vi "RadiusOfCircleThreePoints.vi"(11 "Points":cluster{"X":dbl, "Y":dbl}[](array[cluster])) -> (3 "R":dbl)   [LabVIEW 2017]
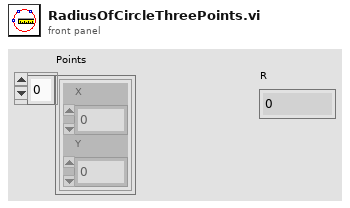
[diagram p1: front panel]
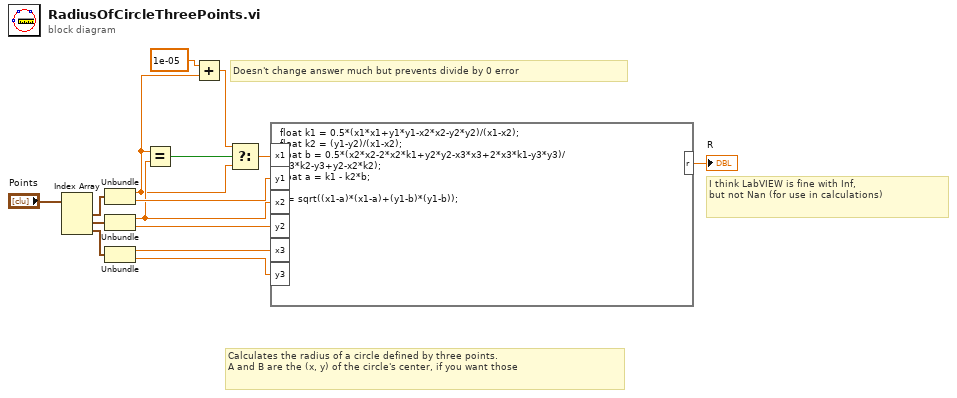
[diagram p0: block diagram]
diagram:
  # "Calculates the radius of a circle defined by three points.\nA and B are the (x, y) of the circle's center, if you want those"
  # "I think LabVIEW is fine with Inf,\nbut not Nan (for use in calculations)"
  # "Doesn't change answer much but prevents divide by 0 error"
  n1 = Index Array(array="Points") -> (element #1=w3:cluster{"X":dbl, "Y":dbl}, element #2=w2:cluster{"X":dbl, "Y":dbl}, element #3=w1:cluster{"X":dbl, "Y":dbl})  [unwired: 3 in]
  n2 = Unbundle(w3) -> ("X"=w8:dbl, "Y"=w15:dbl)
  n3 = Unbundle(w2) -> ("X"=w11:dbl, "Y"=w14:dbl)
  n4 = Unbundle(w1) -> ("X"=w13:dbl, "Y"=w12:dbl)
  n5 = Equal?(x=w8, y=w11) -> (x = y?=w10:bool)
  n6 = Add(x=1e-05, y=w8) -> (x+y=w6:dbl)
  n7 = Select(t=w6, s=w10, f=w8) -> (s? t:f=w9:dbl)
  n8 = formula code="float k1 = 0.5*(x1*x1+y1*y1-x2*x2-y2*y2)/(x1-x2);\nfloat k2 = (y1-y2)/(x1-x2);\nfloat b = 0.5*(x2*x2-2*x2*k1+y2*y2-x3*x3+2*x3*k1-y3*y3)/\n(x3*k2-y3+y2-x2*k2);\nfloat a = k1 - k2*b;\n\nr = sqrt((x1-a)*(x1-a)+(y1-b)*(y1-b));"("x1"=w9, "y1"=w15, "x2"=w11, "y2"=w14, "x3"=w13, "y3"=w12) -> ("r"=→"R":dbl)
